vi "sv_Check for Time and Angle Positions.vi"(0 "data to process":waveform(dbl)[](array[waveform]), 2 "reset?":bool, 11 "error in (no error)":errorcluster, 12 "harmonic":i32=-1) -> (4 "data to process out":waveform(dbl)[](array[waveform]), 6 "time array [s]":dbl[](array[numeric]), 8 "phase array [rad]":dbl[](array[numeric]), 10 "samples/rev":i32, 14 "actual harmonic":i32=-1, 15 "error out":errorcluster)   [LabVIEW 2017, in "SoundVib_ContSweptSine.lvlib"]
uses:
  <vilib>/addons/Sound and Vibration/svt_Continuous Swept Sine/SoundVib_ContSweptSine.lvlib
  <vilib>/addons/Sound and Vibration/svt_Continuous Swept Sine/subVIs/sv_Continuous Swept-Sine Tags.ctl
  <vilib>/addons/Sound and Vibration/svt_Continuous Swept Sine/subVIs/sv_Continuous Swept-Sine Errors.ctl
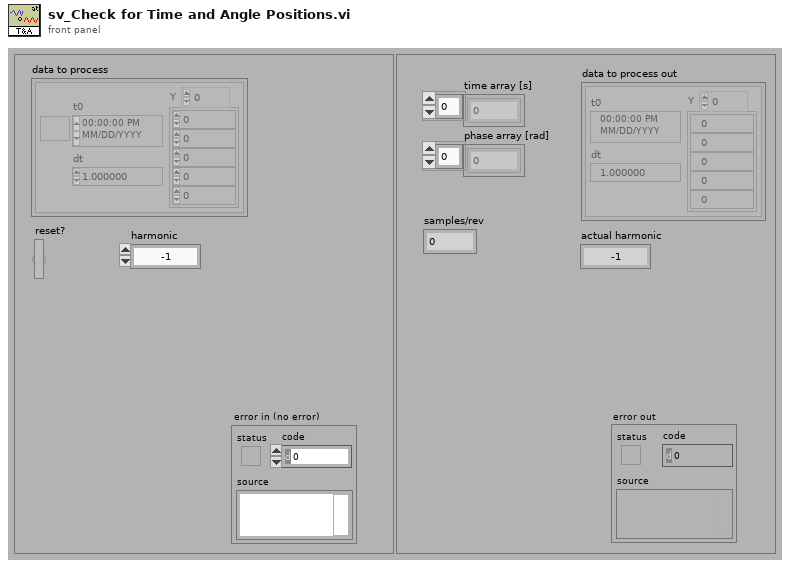
[diagram p1: front panel]
types:
  T1 = typedef "SoundVib_ContSweptSine.lvlib/sv_Continuous Swept-Sine Tags.ctl" = enum16{"samplesPerRevolution", "t2aPositions", "a2tPositions", "evenAngleSignal", "evenAnglePositionInfo", "evenAngleChannelInfo"}
  T2 = typedef "SoundVib_ContSweptSine.lvlib/sv_Continuous Swept-Sine Errors.ctl" = enum16{"Invalid AI sampling rate", "Item not found", "Invalid initial phase"}
  T3 = typedef "SoundVib_Generation.lvlib/sv_Chirp Settings.ctl" = cluster{"amplitude":dbl, "frequency range":cluster{"start (Hz)":dbl, "stop (Hz)":dbl, "frequency spacing":enum16{"Linear", "Logarithmic"}}, "sampling info":cluster{"Fs":dbl, "chirp duration [s]":dbl}, "initial states":cluster{"frequency [Hz]":dbl, "phase [rad]":dbl, "elapsed time [s]":dbl}, "frequency slope":dbl, "maximum harmonic":i32, "prefix len [samples]":cluster{"integer":u32, "fractional":dbl}}
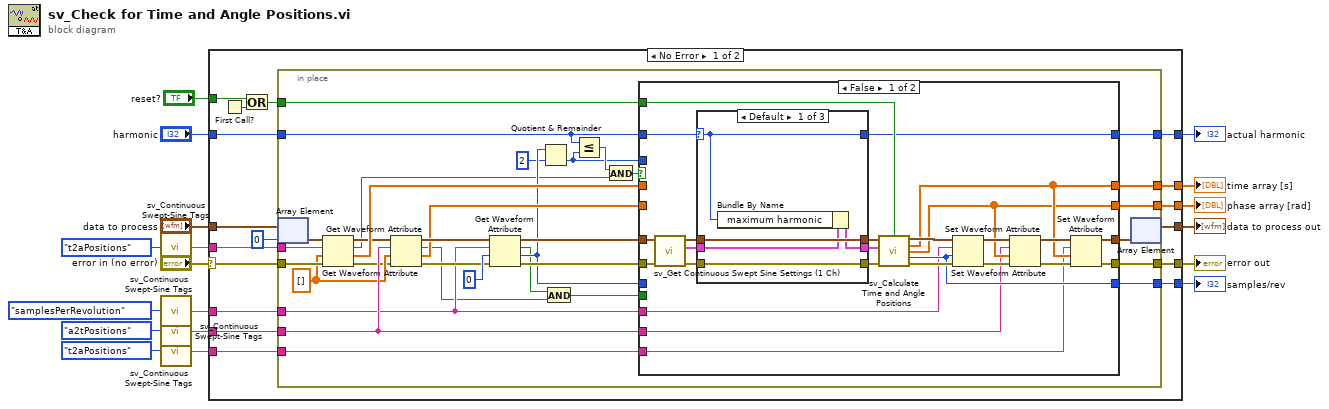
[diagram p0: block diagram]
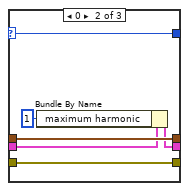
[diagram p2: hidden frame]
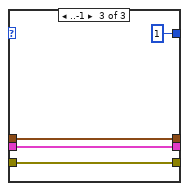
[diagram p3: hidden frame]
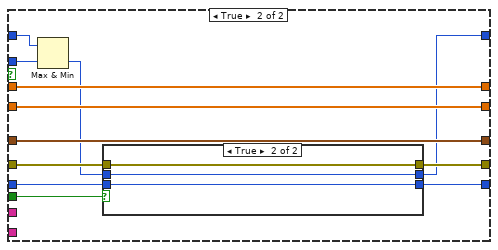
[diagram p4: hidden frame]
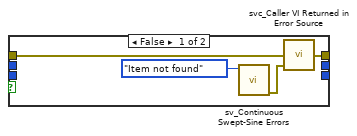
[diagram p5: hidden frame]
diagram:
  n1 = call <vilib>:"sv_Continuous Swept-Sine Tags.vi"("chirp sweep tag selector"=sv_Continuous_Swept-Sine_Tags."t2aPositions" ("chirp sweep error selector")) -> ("Tag"=w10:string)
  n2 = call <vilib>:"sv_Continuous Swept-Sine Tags.vi"("chirp sweep tag selector"=sv_Continuous_Swept-Sine_Tags."samplesPerRevolution" ("chirp sweep error selector")) -> ("Tag"=w5:string)
  n3 = call <vilib>:"sv_Continuous Swept-Sine Tags.vi"("chirp sweep tag selector"=sv_Continuous_Swept-Sine_Tags."a2tPositions" ("chirp sweep error selector")) -> ("Tag"=w4:string)
  n4 = call <vilib>:"sv_Continuous Swept-Sine Tags.vi"("chirp sweep tag selector"=sv_Continuous_Swept-Sine_Tags."t2aPositions" ("chirp sweep error selector")) -> ("Tag"=w3:string)
  n5 = case shown="No Error" "error in (no error)" {
    selector: "error in (no error)" -> [w35 w129]
    tunnel: [w34 w129] -> w17
    tunnel: "data to process" -> [w26 w128]
    tunnel: [w25 w128] -> w15
    tunnel: [w33 _] -> w12
    tunnel: [w32 _] -> w13
    tunnel: "reset?" -> [w29 _]
    tunnel: [w31 _] -> w11
    tunnel: w10 -> [w27 _]
    tunnel: w5 -> [w24 _]
    tunnel: w4 -> [w23 _]
    tunnel: w3 -> [w22 _]
    tunnel: "harmonic" -> [w21 _]
    tunnel: [w20 _] -> w1
    frame No Error {
      n6 = First Call?() -> (First Call?: T/F=w28:bool)
      n7 = Or(x=w29, y=w28) -> (x .or. y?=w30:bool)
      n8 = in-place {
        in-place-border: w35 -> [w68]
        in-place-border: [w67] -> w34
        in-place-border: [w66] -> w33
        in-place-border: [w64] -> w32
        in-place-border: [w63] -> w31
        in-place-border: w30 -> [w62]
        in-place-border: w27 -> [w61]
        in-place-border: w24 -> [w46]
        in-place-border: w23 -> [w55]
        in-place-border: w22 -> [w58]
        in-place-border: w21 -> [w41]
        in-place-border: [w57] -> w20
        w54 = dbl[] [] ("Array")
        n9 = in-place-array #1(w26, 0) -> (w60:waveform(dbl))
        n10 = Get Waveform Attribute(4:w68, 5:w54, 6:w61, 7:w60) -> (0:w53:errorcluster, 1:w65:dbl[], 2:w38:bool, 3:w56:waveform(dbl))
        n11 = Get Waveform Attribute(4:w53, 5:w54, 6:w55, 7:w56) -> (0:w50:errorcluster, 1:w47:dbl[], 2:w43:bool, 3:w51:waveform(dbl))
        n12 = Get Waveform Attribute(4:w50, 5:0 ("samples/rev"), 6:w46, 7:w51) -> (0:w48:errorcluster, 1:w45:i32, 2:w44:bool, 3:w49:waveform(dbl))
        n13 = Quotient & Remainder(x=w45, y=2) -> (floor(x/y)=w37:i32)  [unwired: 1 out]
        n14 = And(x=w44, y=w43) -> (x .and. y?=w42:bool)
        n15 = Less Or Equal?(x=w41, y=w37) -> (x <= y?=w40:bool)
        n16 = And(x=w40, y=w38) -> (x .and. y?=w39:bool)
        n17 = case shown="False" w39 {
          tunnel: w48 -> [w84 w115]
          tunnel: [w87 w120] -> w67
          tunnel: w49 -> [w83 w116]
          tunnel: [w80 w118] -> w66
          tunnel: w65 -> [_ w119]
          tunnel: [w81 w119] -> w64
          tunnel: w62 -> [w86 _]
          tunnel: [w90 w109] -> w63
          tunnel: [w85 w116] -> w59
          tunnel: w46 -> [w79 _]
          tunnel: w55 -> [w78 _]
          tunnel: w58 -> [w77 _]
          tunnel: w41 -> [w76 w114]
          tunnel: [w69 w111] -> w57
          tunnel: w47 -> [_ w118]
          tunnel: w45 -> [_ w110]
          tunnel: w42 -> [_ w117]
          tunnel: w37 -> [_ w113]
          frame False {
            n18 = call <vilib>:"sv_Get Continuous Swept Sine Settings (1 Ch).vi"("error in (no error)"=w84, "waveform"=w83) -> ("error out"=w70:errorcluster, "chirp settings out"=w73:T3, "same waveform"=w75:waveform(dbl))  [unwired: 7 in]
            n19 = case shown="Default" w76 {
              selector: w76 -> [w94 w100 _]
              tunnel: w75 -> [w98 w104 w108]
              tunnel: [w98 w104 w108] -> w74
              tunnel: w73 -> [w96 w102 w106]
              tunnel: [w95 w101 w106] -> w72
              tunnel: [w97 w103 w107] -> w71
              tunnel: w70 -> [w97 w103 w107]
              tunnel: [w94 w100 1 ("maximum harmonic")] -> w69
              frame Default {
                n20 = Bundle By Name(cluster=w96, "maximum harmonic"=w94) -> (w95:T3)
              }
              frame 0 {
                n21 = Bundle By Name(cluster=w102, "maximum harmonic"=1) -> (w101:T3)
              }
              frame ..-1 {
              }
            }
            n22 = call <vilib>:"sv_Calculate Time and Angle Positions.vi"("waveform in"=w74, "reset?"=w86, "chirp settings"=w72, "error in (no error)"=w71) -> ("waveform out"=w82:waveform(dbl), "time array [s]"=w81:dbl[], "phase array [rad]"=w80:dbl[], "samples/rev"=w90:i32, "error out"=w91:errorcluster)  [unwired: 7 in]
            n23 = Set Waveform Attribute(4:w91, 5:w90, 6:w79, 7:w82) -> (0:w92:errorcluster, 3:w93:waveform(dbl))  [unwired: 1 out]
            n24 = Set Waveform Attribute(4:w92, 5:w80, 6:w78, 7:w93) -> (0:w89:errorcluster, 3:w88:waveform(dbl))  [unwired: 1 out]
            n25 = Set Waveform Attribute(4:w89, 5:w81, 6:w77, 7:w88) -> (0:w87:errorcluster, 3:w85:waveform(dbl))  [unwired: 1 out]
          }
          frame True {
            n26 = Max & Min(x=w114, y=w113) -> (min(x,y)=w112:i32)  [unwired: 1 out]
            n27 = case shown="True" w117 {
              tunnel: w115 -> [w123 w127]
              tunnel: [w122 w127] -> w120
              tunnel: w112 -> [_ w126]
              tunnel: [_ w126] -> w111
              tunnel: w110 -> [_ w125]
              tunnel: [_ w125] -> w109
              frame False {
                n28 = call <vilib>:"sv_Continuous Swept-Sine Errors.vi"("continuous swept-sine error"=sv_Continuous_Swept-Sine_Errors."Item not found" ("chirp sweep error selector")) -> ("error out"=w124:errorcluster)  [unwired: 10 in]
                n29 = call <vilib>:"svc_Caller VI Returned in Error Source.vi"("warning input to caller"=w124, "error in (no error)"=w123) -> ("error out"=w122:errorcluster)  [unwired: 3 in]
              }
              frame True {
              }
            }
          }
        }
        n30 = in-place-array #1(w59) -> (w25:waveform(dbl)[])  [unwired: 1 out]
      }
    }
    frame Error {
    }
  }
  "error out" <- w17
  "data to process out" <- w15
  "time array [s]" <- w13
  "phase array [rad]" <- w12
  "samples/rev" <- w11
  "actual harmonic" <- w1
